vi "DoCreateError.vi"(5 "MergeErrors":bool, 6 "AdditionalText":string, 7 "Data":variant, 8 "ErrorIn":errorcluster caption="Error In", 9 "Text":string, 10 "ErrorCode":i32, 11 "Object in":refnum<class "ErrorCreationTAF.lvclass"> caption="Object In") -> (0 "ErrorOut":errorcluster caption="Error Out", 3 "Object out":refnum<class "ErrorCreationTAF.lvclass"> caption="Object Out")   [LabVIEW 2021, in "ErrorCreationTAF.lvclass"]
uses:
  ErrorCreationTAF.lvclass
  fec1759e-50a6-418f-9aeb-0391d960c39c.vi
  eaf0681e-e464-4b3a-95e7-fa23abfdab0d.vi
  <vilib>/JDP Science/JSONtext/Variant to JSON Text.vi
  <vilib>/JDP Science/JSONtext/LVClass Serializer/JSONtext LVClass Serializer.lvclass
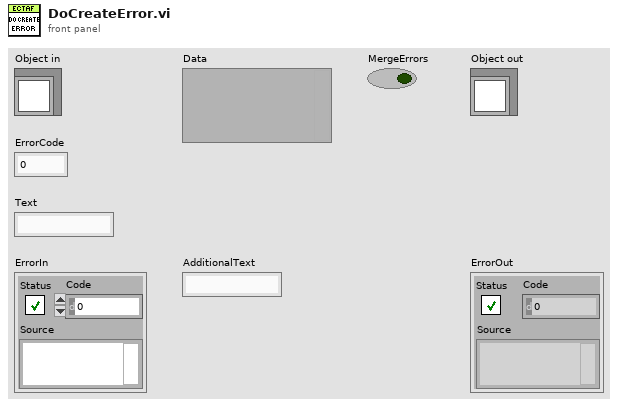
[diagram p1: front panel]
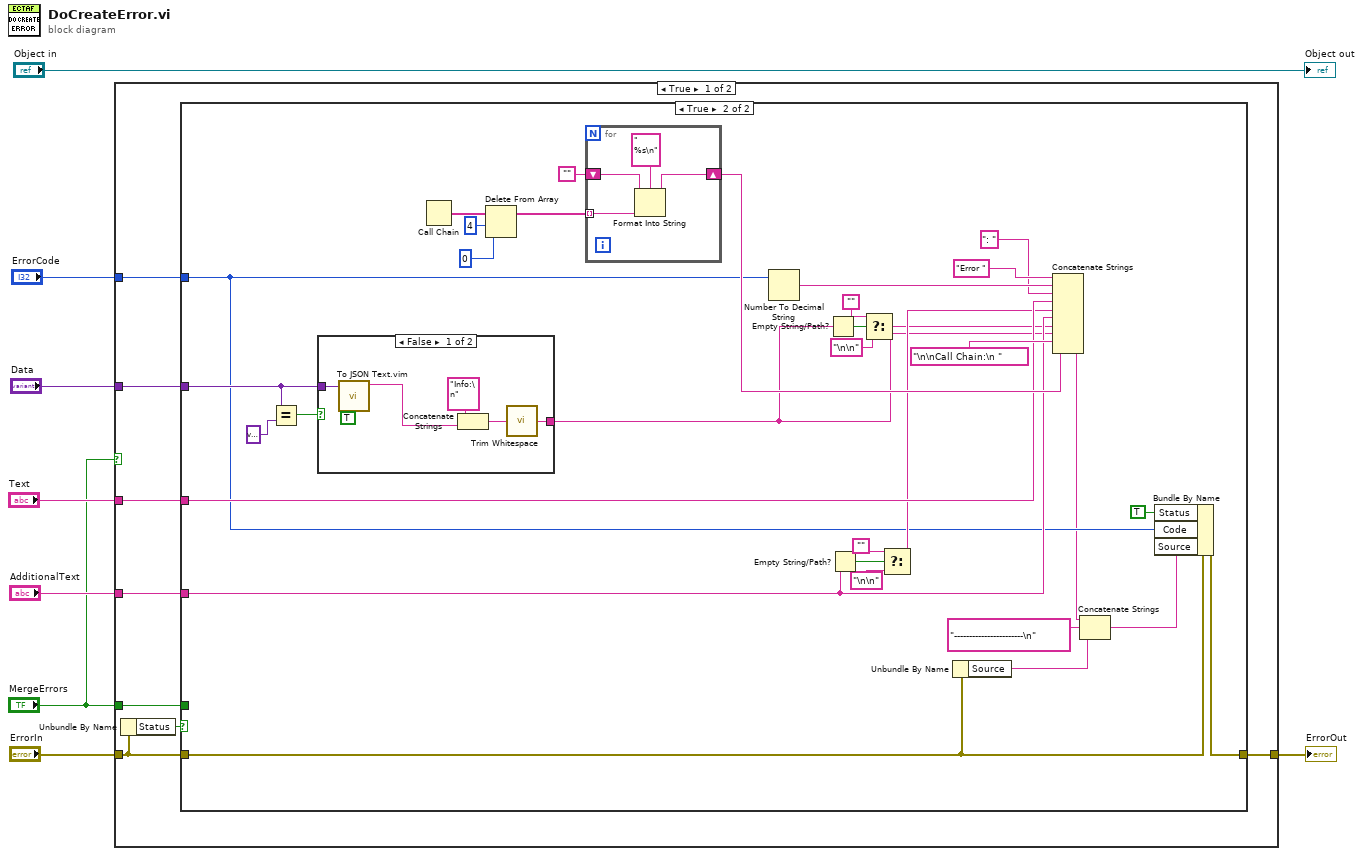
[diagram p0: block diagram]
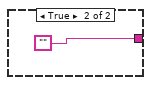
[diagram p3: hidden frame]
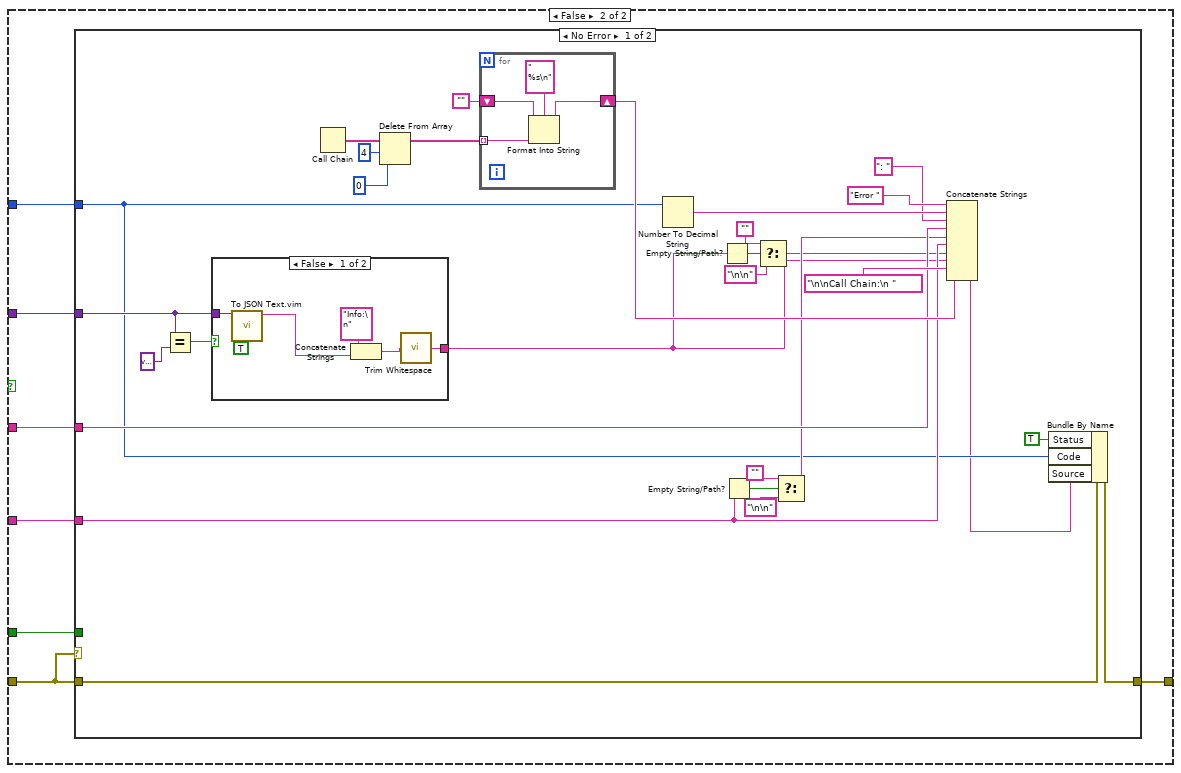
[diagram p4: hidden frame]
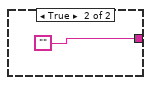
[diagram p5: hidden frame]
diagram:
  n1 = case shown="True" "MergeErrors" {
    tunnel: [w16 w67] -> w8
    tunnel: "Data" -> [w15 w66]
    tunnel: "Text" -> [w14 w65]
    tunnel: "AdditionalText" -> [w13 w64]
    tunnel: "ErrorCode" -> [w12 w63]
    tunnel: "MergeErrors" -> [w11 w62]
    tunnel: "ErrorIn" -> [w10 w61]
    frame True {
      n2 = Unbundle By Name(w10) -> ("Status"=w9:bool)
      n3 = case shown="True" w9 {
        tunnel: w10 -> [w17 w18]
        tunnel: [w17 w49] -> w16
        tunnel: w15 -> [_ w48]
        tunnel: w14 -> [_ w34]
        tunnel: w13 -> [_ w28]
        tunnel: w12 -> [_ w23]
        tunnel: w11 -> [_ _]
        frame False {
        }
        frame True {
          n4 = Equal?(x=w48, y=variant) -> (x = y?=w45:bool)
          n5 = case shown="False" w45 {
            tunnel: [w57 ""] -> w26
            tunnel: w48 -> [w56 _]
            frame False {
              n6 = call "To JSON Text.vim"("Pretty Print?"=TRUE, "Anything"=w56) -> ("<JSON>"=w54:string)  [unwired: 8 in, 1 out]
              n7 = Concatenate Strings("Info:\n" ("string"), w54) -> (w59:string)
              n8 = call <vilib>:"Trim Whitespace.vi"("string"=w59) -> ("trimmed string"=w57:string)  [unwired: 1 in]
            }
            frame True {
            }
          }
          n9 = Call Chain() -> (call chain=w43:string[])
          n10 = Delete From Array(array=w43, length=4, index=0 ("length")) -> (array with subset deleted=w42:string[])  [unwired: 1 out]
          n11 = for {
            tunnel: w42 -> [w53] mode=indexing
            shift-right: [w51] -> w35
            shift-left: "" -> [w52]
            n12 = Format Into String(format string="  %s\n", initial string=w52, w53) -> (resulting string=w51:string)  [unwired: 1 in, 1 out]
          }
          n13 = Number To Decimal String(number=w23) -> (decimal integer string=w38:string)  [unwired: 1 in]
          n14 = Empty String/Path?(string/path=w26) -> (empty?=w30:bool)
          n15 = Empty String/Path?(string/path=w28) -> (empty?=w33:bool)
          n16 = Select(t="", s=w30, f="\n\n") -> (s? t:f=w27:string)
          n17 = Select(t="", s=w33, f="\n\n") -> (s? t:f=w29:string)
          n18 = Unbundle By Name(w18) -> ("Source"=w22:string)
          n19 = Concatenate Strings("Error " ("format string"), w38, ": " ("format string"), w34, w29, w28, w27, w26, "\n\nCall Chain:\n " ("format string"), w35) -> (w20:string)
          n20 = Concatenate Strings(w20, "-----------------------\n" ("string"), w22) -> (w19:string)
          n21 = Bundle By Name(cluster=w18, "Status"=TRUE ("status"), "Code"=w23, "Source"=w19) -> (w49:errorcluster)
        }
      }
    }
    frame False {
      n22 = case shown="No Error" w61 {
        tunnel: w61 -> [w68 w108]
        tunnel: [w96 w108] -> w67
        tunnel: w66 -> [w95 _]
        tunnel: w65 -> [w81 _]
        tunnel: w64 -> [w75 _]
        tunnel: w63 -> [w70 _]
        tunnel: w62 -> [_ _]
        frame No Error {
          n23 = Equal?(x=w95, y=variant) -> (x = y?=w92:bool)
          n24 = case shown="False" w92 {
            tunnel: [w106 ""] -> w73
            tunnel: w95 -> [w102 _]
            frame False {
              n25 = call "To JSON Text.vim"("Pretty Print?"=TRUE, "Anything"=w102) -> ("<JSON>"=w103:string)  [unwired: 8 in, 1 out]
              n26 = Concatenate Strings("Info:\n" ("string"), w103) -> (w101:string)
              n27 = call <vilib>:"Trim Whitespace.vi"("string"=w101) -> ("trimmed string"=w106:string)  [unwired: 1 in]
            }
            frame True {
            }
          }
          n28 = Call Chain() -> (call chain=w90:string[])
          n29 = Delete From Array(array=w90, length=4, index=0 ("length")) -> (array with subset deleted=w89:string[])  [unwired: 1 out]
          n30 = for {
            tunnel: w89 -> [w100] mode=indexing
            shift-right: [w98] -> w82
            shift-left: "" -> [w99]
            n31 = Format Into String(format string="  %s\n", initial string=w99, w100) -> (resulting string=w98:string)  [unwired: 1 in, 1 out]
          }
          n32 = Number To Decimal String(number=w70) -> (decimal integer string=w85:string)  [unwired: 1 in]
          n33 = Empty String/Path?(string/path=w73) -> (empty?=w77:bool)
          n34 = Empty String/Path?(string/path=w75) -> (empty?=w80:bool)
          n35 = Select(t="", s=w77, f="\n\n") -> (s? t:f=w74:string)
          n36 = Select(t="", s=w80, f="\n\n") -> (s? t:f=w76:string)
          n37 = Concatenate Strings("Error " ("format string"), w85, ": " ("format string"), w81, w76, w75, w74, w73, "\n\nCall Chain:\n " ("format string"), w82) -> (w69:string)
          n38 = Bundle By Name(cluster=w68, "Status"=TRUE ("status"), "Code"=w70, "Source"=w69) -> (w96:errorcluster)
        }
        frame Error {
        }
      }
    }
  }
  "ErrorOut" <- w8
  "Object out" <- "Object in"
